vi "Change Directory Permissions I16.vi"(0 "path":path=path "C:/Program Files (x86)/National Instruments/RT Images/User Components", 5 "user":T1={"read"=TRUE, "write"=FALSE, "execute"=TRUE}, 7 "group":T1={"read"=TRUE, "write"=FALSE, "execute"=TRUE}, 9 "others":T1={"read"=TRUE, "write"=FALSE, "execute"=TRUE}, 11 "error in":errorcluster, 12 "Action (Get)":enum16{"Get", "Scan", "Set", "Restore"}(ring)) -> (4 "path out":path, 6 "permissions":i16, 15 "error out":errorcluster)   [LabVIEW 2015]
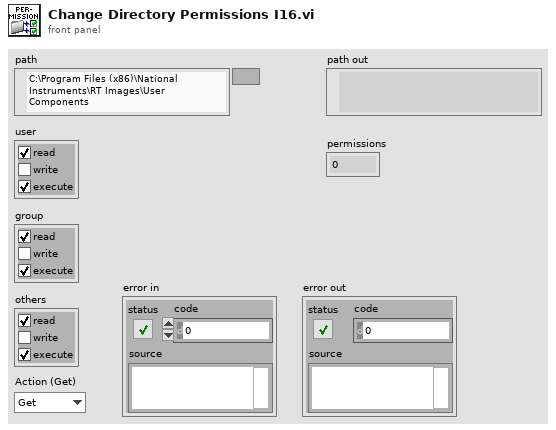
[diagram p1: front panel]
types:
  T1 = cluster{"read":bool, "write":bool, "execute":bool}
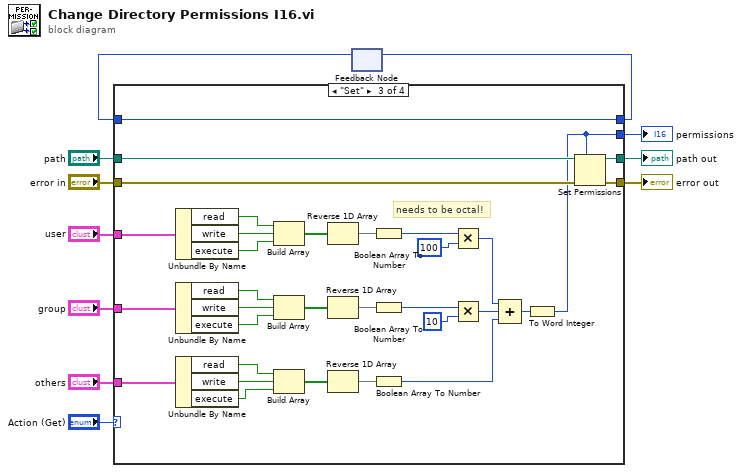
[diagram p0: block diagram]
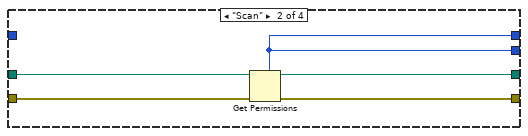
[diagram p3: hidden frame]
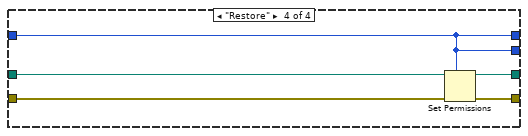
[diagram p4: hidden frame]
diagram:
  n1 = feedback #1() -> (w8:i16)  [unwired: 1 in]
  n2 = case shown="\"Set\"" "Action (Get)" {
    tunnel: "path" -> [w14 w19 w51 w56]
    tunnel: "error in" -> [w13 w18 w50 w55]
    tunnel: [w12 w15 w20 w52] -> w2
    tunnel: w8 -> [w12 _ w21 w52]
    tunnel: "user" -> [_ _ w28 _]
    tunnel: "group" -> [_ _ w27 _]
    tunnel: "others" -> [_ _ w26 _]
    tunnel: [w14 w16 w24 w54] -> w3
    tunnel: [w13 w17 w23 w53] -> w4
    tunnel: [w12 w15 w21 w52] -> w1
    frame "Get", Default {
    }
    frame "Scan" {
      n3 = Get Permissions(8:w18, 11:w19) -> (0:w17:errorcluster, 3:w16:path, 5:w15:i16)  [unwired: 2 out]
    }
    frame "Set" {
      # "needs to be octal!"
      n4 = Unbundle By Name(w28) -> ("read"=w36:bool, "write"=w37:bool, "execute"=w38:bool)
      n5 = Unbundle By Name(w27) -> ("read"=w40:bool, "write"=w41:bool, "execute"=w42:bool)
      n6 = Unbundle By Name(w26) -> ("read"=w43:bool, "write"=w44:bool, "execute"=w22:bool)
      n7 = Build Array(w36, w37, w38) -> (w39:bool[])
      n8 = Build Array(w40, w41, w42) -> (w45:bool[])
      n9 = Build Array(w43, w44, w22) -> (w46:bool[])
      n10 = Reverse 1D Array(array=w39) -> (reversed array=w49:bool[])
      n11 = Reverse 1D Array(array=w45) -> (reversed array=w48:bool[])
      n12 = Reverse 1D Array(array=w46) -> (reversed array=w47:bool[])
      n13 = Boolean Array To Number(Boolean array=w49) -> (number=w29:u32)
      n14 = Boolean Array To Number(Boolean array=w48) -> (number=w31:u32)
      n15 = Boolean Array To Number(Boolean array=w47) -> (number=w35:u32)
      n16 = Multiply(x=w29, y=u32 100) -> (x*y=w33:u32)
      n17 = Multiply(x=w31, y=u32 10) -> (x*y=w34:u32)
      n18 = Compound Arithmetic op=ADD(w33, w34, w35) -> (w25:u32)
      n19 = To Word Integer(number=w25) -> (16bit integer=w20:i16)
      n20 = Set Permissions(7:w20, 8:w50, 11:w51) -> (0:w23:errorcluster, 3:w24:path)  [unwired: 2 in]
    }
    frame "Restore" {
      n21 = Set Permissions(7:w52, 8:w55, 11:w56) -> (0:w53:errorcluster, 3:w54:path)  [unwired: 2 in]
    }
  }
  "error out" <- w4
  "path out" <- w3
  "permissions" <- w2
  n22 = feedback-in #1(w1) -> ()
